vi "percentdonev2.vi"(1 "input tone end power (dBm)":dbl[](array[numeric]), 2 "Array":dbl[](array[numeric]), 3 "input tone start power (dBm)":dbl[](array[numeric])) -> (0 "Numeric":dbl)   [LabVIEW 2009]
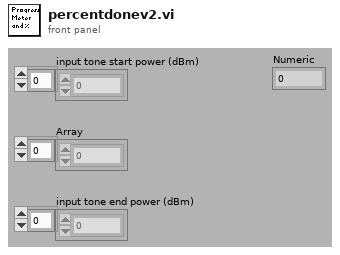
[diagram p1: front panel]
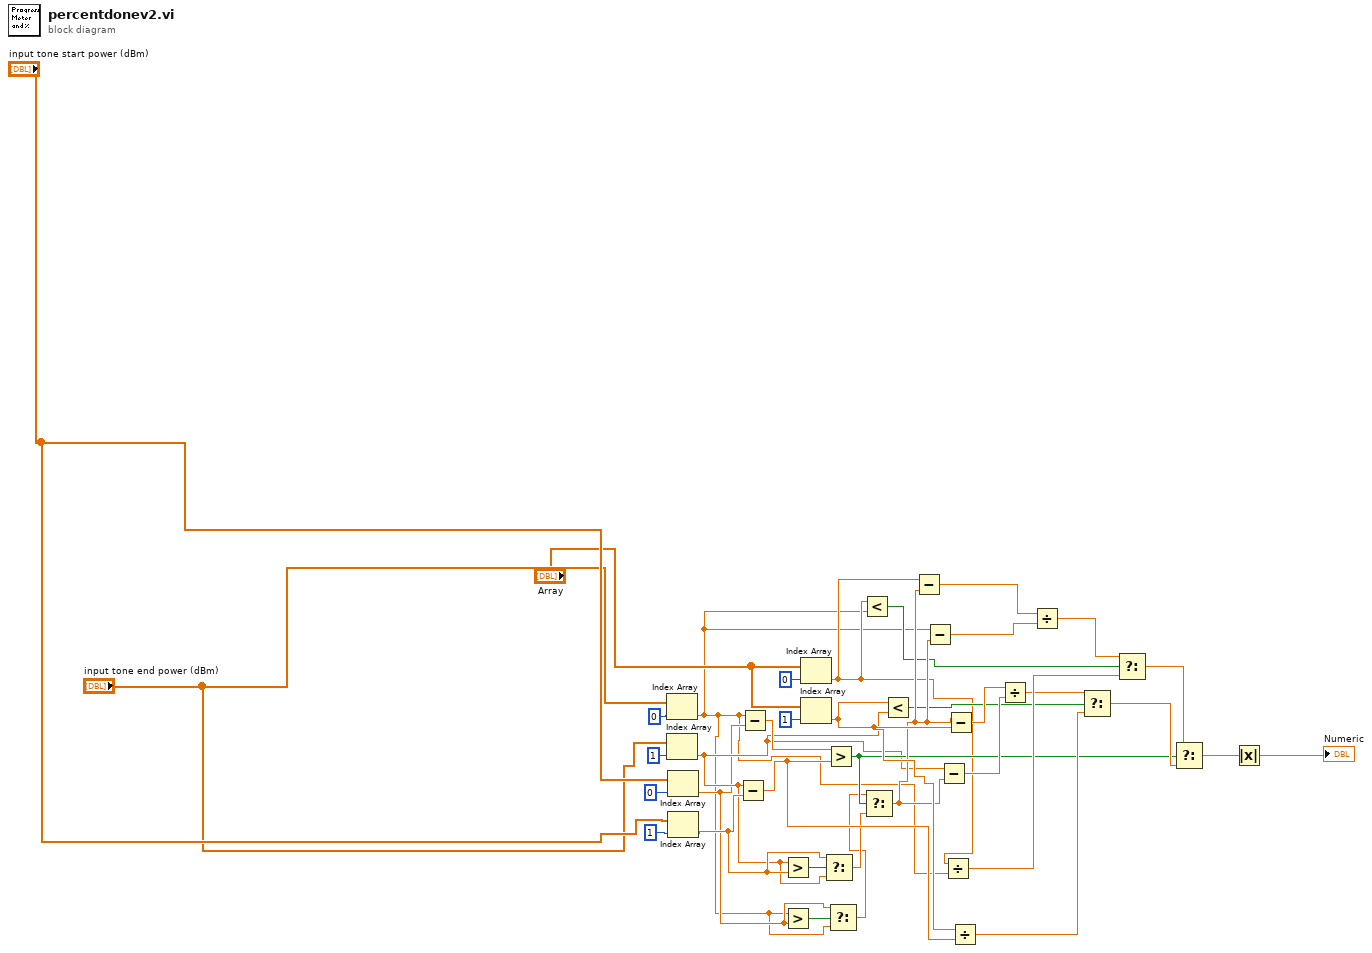
[diagram p0: block diagram]
diagram:
  n1 = Index Array(array="input tone end power (dBm)", index=0) -> (element=w6:dbl)
  n2 = Index Array(array="input tone end power (dBm)", index=1) -> (element=w9:dbl)
  n3 = Index Array(array="input tone start power (dBm)", index=0) -> (element=w7:dbl)
  n4 = Index Array(array="input tone start power (dBm)", index=1) -> (element=w10:dbl)
  n5 = Subtract(x=w9, y=w10) -> (x-y=w33:dbl)
  n6 = Subtract(x=w6, y=w7) -> (x-y=w20:dbl)
  n7 = Greater?(x=w9, y=w10) -> (0:w11:bool)
  n8 = Greater?(x=w6, y=w7) -> (0:w8:bool)
  n9 = Index Array(array="Array", index=0) -> (element=w12:dbl)
  n10 = Index Array(array="Array", index=1) -> (element=w32:dbl)
  n11 = Select(t=w10, s=w11, f=w9) -> (s? t:f=w5:dbl)
  n12 = Greater?(x=w20, y=w33) -> (0:w21:bool)
  n13 = Select(t=w7, s=w8, f=w6) -> (s? t:f=w4:dbl)
  n14 = Less?(x=w12, y=w6) -> (x < y?=w22:bool)
  n15 = Select(t=w4, s=w21, f=w5) -> (s? t:f=w26:dbl)
  n16 = Less?(x=w32, y=w9) -> (x < y?=w23:bool)
  n17 = Subtract(x=w12, y=w26) -> (x-y=w3:dbl)
  n18 = Subtract(x=w6, y=w26) -> (x-y=w24:dbl)
  n19 = Subtract(x=w9, y=w26) -> (x-y=w27:dbl)
  n20 = Divide(x=w12, y=w6) -> (x/y=w34:dbl)
  n21 = Subtract(x=w26, y=w32) -> (x-y=w28:dbl)
  n22 = Divide(x=w32, y=w33) -> (x/y=w35:dbl)
  n23 = Divide(x=w28, y=w27) -> (x/y=w29:dbl)
  n24 = Divide(x=w3, y=w24) -> (x/y=w25:dbl)
  n25 = Select(t=w29, s=w23, f=w35) -> (s? t:f=w31:dbl)
  n26 = Select(t=w25, s=w22, f=w34) -> (s? t:f=w30:dbl)
  n27 = Select(t=w30, s=w21, f=w31) -> (s? t:f=w2:dbl)
  n28 = Absolute Value(x=w2) -> (abs(x)=→"Numeric":dbl)
